vi "1D Histogram or PDF, weighted_PN.vi"(0 "Nbins":i32, 3 "Mean shift":bool, 4 "mean":dbl, 7 "max":dbl, 8 "Current block no.":i32, 9 "min":dbl, 11 "Shift SumW in":dbl, 12 "PDF":bool=TRUE, 13 "Shift PDF in":dbl[](array[numeric]), 16 "1D data":dbl[](array[numeric]), 18 "Weights":dbl[](array[numeric])) -> (20 "1D histogram or PDF":dbl[](array[numeric]), 22 "bin centre vals.":dbl[](array[numeric]), 24 "bin width":dbl, 26 "Shift SumW out":dbl, 27 "Shift PDF out":dbl[](array[numeric]))   [LabVIEW 2011]
panel:
  out "1D histogram or PDF":cluster{"UbinC":dbl[], dbl[]}(graph)
  # "N.B. The values of Umax, Umin, Umean MUST be those of the ENTIRE dataset (i.e. all blocks) otherwise this routine will be inconsistent."
  # "Paul Nathan 03/10/2012"
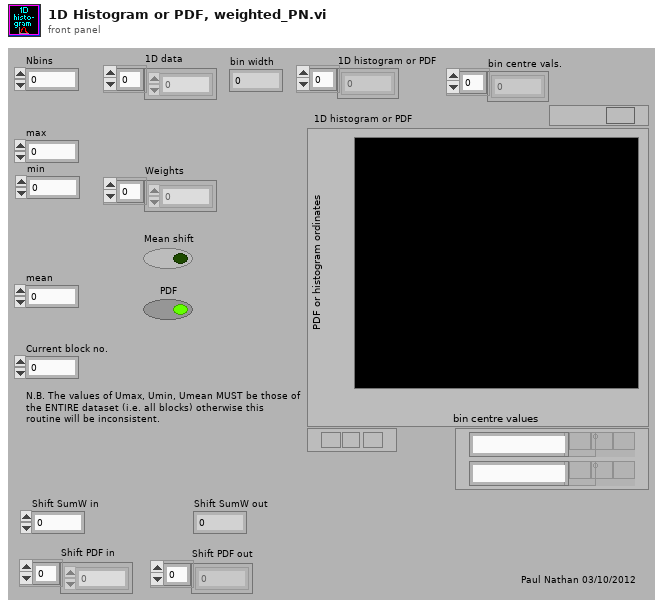
[diagram p1: front panel]
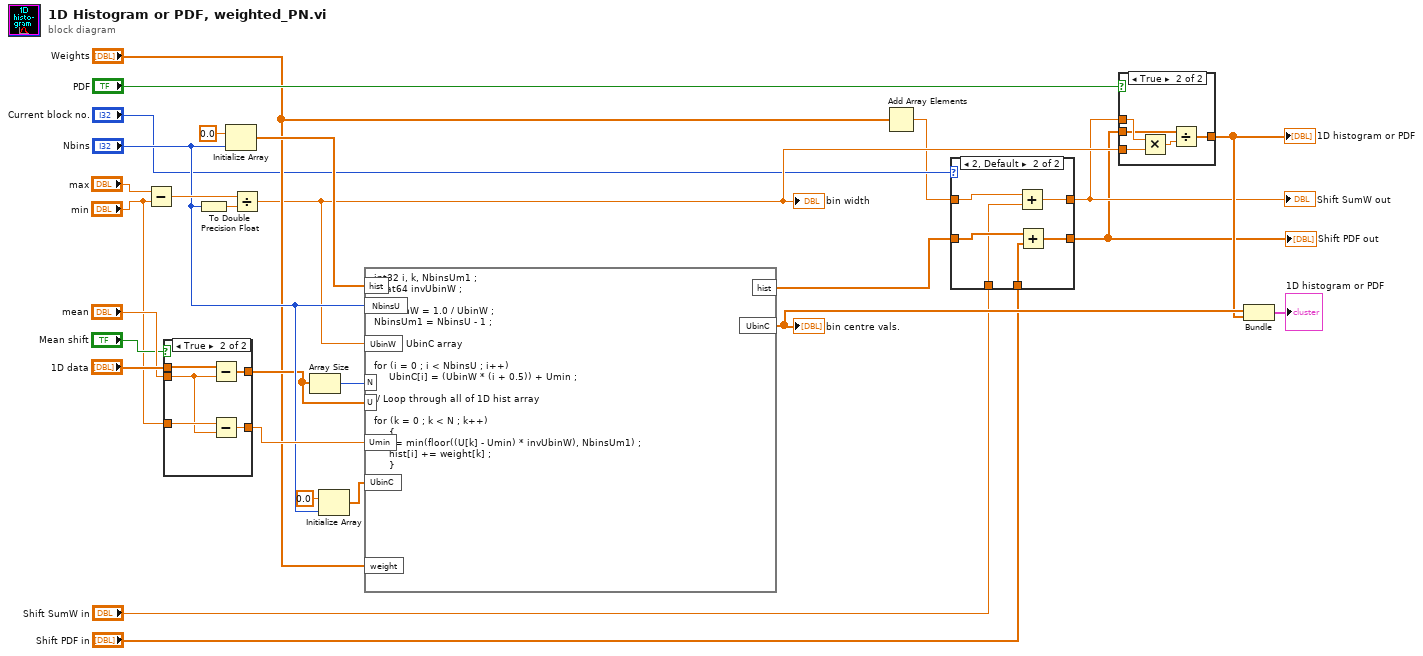
[diagram p0: block diagram]
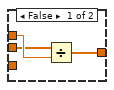
[diagram p3: hidden frame]
diagram:
  n1 = Subtract(x="max", y="min") -> (x-y=w20:dbl)
  n2 = case shown="True" "Mean shift" {
    tunnel: "1D data" -> [w30 w35]
    tunnel: "mean" -> [_ w32]
    tunnel: [w30 w34] -> w16
    tunnel: "min" -> [w29 w33]
    tunnel: [w29 w31] -> w19
    frame False {
    }
    frame True {
      n3 = Subtract(x=w35, y=w32) -> (x-y=w34:dbl[])
      n4 = Subtract(x=w33, y=w32) -> (x-y=w31:dbl)
    }
  }
  n5 = To Double Precision Float(number="Nbins") -> (double precision float=w28:dbl)
  n6 = Initialize Array(0.0 ("element"), "Nbins") -> (w23:dbl[])
  n7 = Divide(x=w20, y=w28) -> (x/y=w11:dbl)
  "bin width" <- w11
  n8 = Array Size(array=w16) -> (size(s)=w13:i32)
  n9 = Initialize Array(0.0 ("element"), "Nbins") -> (w15:dbl[])
  n10 = formula code="int32 i, k, NbinsUm1 ;\nfloat64 invUbinW ;\n\ninvUbinW = 1.0 / UbinW ;\nNbinsUm1 = NbinsU - 1 ;\n\n// Calc UbinC array\n\nfor (i = 0 ; i < NbinsU ; i++)\n     UbinC[i] = (UbinW * (i + 0.5)) + Umin ;\n\n// Loop through all of 1D hist array \n\nfor (k = 0 ; k < N ; k++)\n     {\n     i = min(floor((U[k] - Umin) * invUbinW), NbinsUm1) ;\n     hist[i] += weight[k] ;\n     }"("NbinsU"="Nbins", "N"=w13, "UbinW"=w11, "hist"=w23, "Umin"=w19, "UbinC"=w15, "U"=w16, "weight"="Weights") -> ("hist"=w6:dbl[], "UbinC"=w10:dbl[])
  "bin centre vals." <- w10
  n11 = Add Array Elements(numeric array="Weights") -> (sum=w5:dbl)
  n12 = case shown="2, Default" "Current block no." {
    tunnel: [w37 w42] -> w3
    tunnel: w6 -> [w37 w41]
    tunnel: w5 -> [w36 w40]
    tunnel: [w36 w43] -> w4
    tunnel: "Shift PDF in" -> [_ w39]
    tunnel: "Shift SumW in" -> [_ w38]
    frame 1 {
    }
    frame 2, Default {
      n13 = Add(x=w40, y=w38) -> (x+y=w43:dbl)
      n14 = Add(x=w41, y=w39) -> (x+y=w42:dbl[])
    }
  }
  "Shift PDF out" <- w3
  "Shift SumW out" <- w4
  n15 = case shown="True" "PDF" {
    tunnel: w11 -> [_ w50]
    tunnel: w4 -> [w46 w51]
    tunnel: w3 -> [w45 w49]
    tunnel: [w44 w47] -> w9
    frame False {
      n16 = Divide(x=w45, y=w46) -> (x/y=w44:dbl[])
    }
    frame True {
      n17 = Multiply(x=w51, y=w50) -> (x*y=w48:dbl)
      n18 = Divide(x=w49, y=w48) -> (x/y=w47:dbl[])
    }
  }
  "1D histogram or PDF" <- w9
  n19 = Bundle("UbinC"=w10, w9) -> (→"1D histogram or PDF":cluster{"UbinC":dbl[], dbl[]})  [unwired: 1 out]
